vi "ExampleReader.vi"() -> ()   [LabVIEW 2011]
uses:
  Reader/readType.ctl
  HelperVIs/EStopAction.ctl
  Reader/NetworkStreamReader.lvclass
panel:
  out "Connected?":bool
  out "Cluster":T1
  out "Iteration Time Stamp":timestamp
  out "OCU Time Stamp":timestamp
  in  "stop":bool
  in  "Read Type":T2=enum."Most current"
  in  "Loop delay (ms)":u32=10
  out "element":variant
  out "data":i32
  # "Note: writer is running at 50 ms"
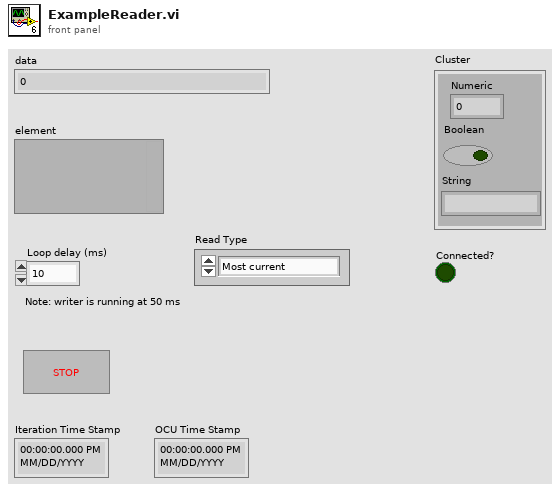
[diagram p1: front panel]
types:
  T1 = cluster{"Numeric":dbl, "Boolean":bool, "String":string}
  T2 = typedef "NetworkStreamReader.lvclass/readType.ctl" = enum16{"Next in buffer", "Most current"}
  T3 = typedef "EStopAction.ctl" = enum16{"Get", "Set"}
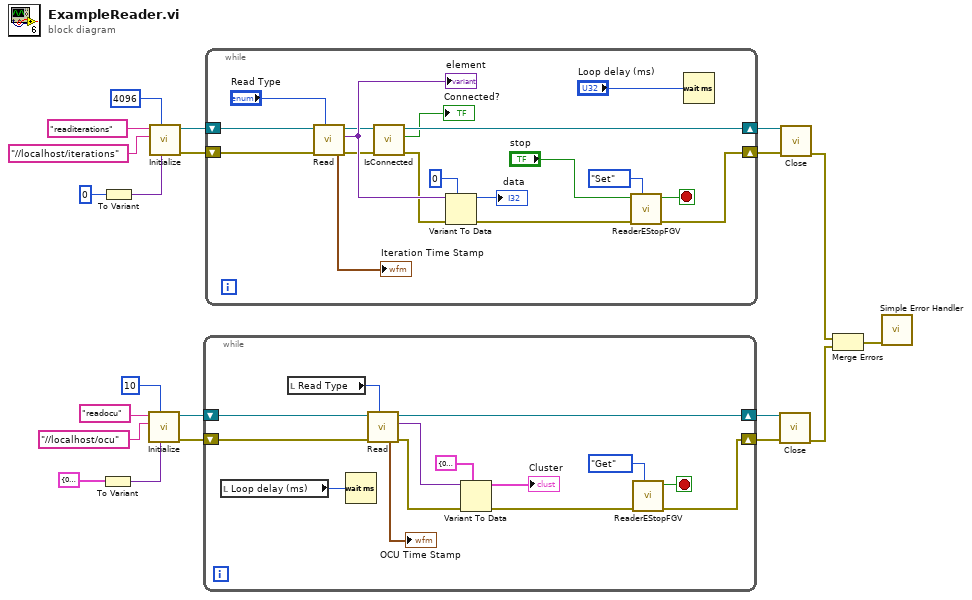
[diagram p0: block diagram]
diagram:
  n1 = To Variant(anything=T1 {"Numeric"=0.0, "Boolean"=FALSE, "String"=""} ("Cluster")) -> (Variant=w14:variant)
  n2 = To Variant(anything=0) -> (Variant=w15:variant)
  n3 = call "Initialize.vi"("Default return"=w14, "reader buffer size"=10 ("writer buffer size"), "writer url"="//localhost/ocu", "reader name"="readocu") -> ("error out"=w9:errorcluster, "NetworkStreamWriter out"=w11:refnum<class "NetworkStreamReader.lvclass">)  [unwired: 6 in]
  n4 = call "Initialize.vi"("Default return"=w15, "reader buffer size"=4096 ("writer buffer size"), "writer url"="//localhost/iterations", "reader name"="readiterations") -> ("error out"=w21:errorcluster, "NetworkStreamWriter out"=w19:refnum<class "NetworkStreamReader.lvclass">)  [unwired: 6 in]
  n5 = while {
    shift-right: [w33] -> w13
    shift-left: w11 -> [w35]
    shift-right: [w22] -> w12
    shift-left: w9 -> [w34]
    stop <- w23 stop-if-true
    n6 = local read "Loop delay (ms)"() -> (w30:u32)
    n7 = local read "Read Type"() -> (w31:T2)
    n8 = Wait (ms)(milliseconds to wait=w30) -> ()  [unwired: 1 out]
    n9 = call "Read.vi"("Read Type"=w31, "error in (no error)"=w34, "NetworkStreamReader in"=w35) -> ("error out"=w29:errorcluster, "element"=w32:variant, "NetworkStreamReader out"=w33:refnum<class "NetworkStreamReader.lvclass">, "Time Stamp"=→"OCU Time Stamp":timestamp)  [unwired: 4 in, 1 out]
    n10 = Variant To Data(error in=w29, type=T1 {"Numeric"=0.0, "Boolean"=FALSE, "String"=""} ("Cluster"), Variant=w32) -> (data=→"Cluster":T1, error out=w24:errorcluster)
    n11 = call "ReaderEStopFGV.vi"("E-Stop Action"=EStopAction."Get", "Error In"=w24) -> ("Error Out"=w22:errorcluster, "E-Stop Out"=w23:bool)  [unwired: 8 in]
  }
  n12 = while {
    shift-right: [w37] -> w17
    shift-left: w19 -> [w53]
    shift-right: [w41] -> w18
    shift-left: w21 -> [w52]
    stop <- w42 stop-if-true
    n13 = call "Read.vi"("Read Type"="Read Type", "error in (no error)"=w52, "NetworkStreamReader in"=w53) -> ("error out"=w39:errorcluster, "element"=w51:variant, "NetworkStreamReader out"=w40:refnum<class "NetworkStreamReader.lvclass">, "Time Stamp"=→"Iteration Time Stamp":timestamp)  [unwired: 4 in, 1 out]
    "element" <- w51
    n14 = call "IsConnected.vi"("error in (no error)"=w39, "NetworkStreamReader in"=w40) -> ("error out"=w38:errorcluster, "Connected?"=→"Connected?":bool, "NetworkStreamReader out"=w37:refnum<class "NetworkStreamReader.lvclass">)  [unwired: 7 in]
    n15 = Variant To Data(error in=w38, type=0, Variant=w51) -> (data=→"data":i32, error out=w44:errorcluster)
    n16 = call "ReaderEStopFGV.vi"("E-Stop Action"=EStopAction."Set", "Error In"=w44, "E-Stop In"="stop") -> ("Error Out"=w41:errorcluster, "E-Stop Out"=w42:bool)  [unwired: 7 in]
    n17 = Wait (ms)(milliseconds to wait="Loop delay (ms)") -> ()  [unwired: 1 out]
  }
  n18 = call "Close.vi"("error in (no error)"=w12, "NetworkStreamReader in"=w13) -> ("error out"=w7:errorcluster)  [unwired: 9 in]
  n19 = call "Close.vi"("error in (no error)"=w18, "NetworkStreamReader in"=w17) -> ("error out"=w8:errorcluster)  [unwired: 9 in]
  n20 = Merge Errors(w8, w7) -> (w1:errorcluster)
  n21 = call <vilib>:"Simple Error Handler.vi"("error in (no error)"=w1) -> ()  [unwired: 4 in, 5 out]
